vi "Launch Mask.vi"(4 "Pane Color":u32, 6 "Panel State":T1(ring)=enum."Standard", 8 "Error in":errorcluster caption="Error in (no error)", 9 "Bounds":T2, 10 "Panel Transparency":u8=60) -> (0 "Error out":errorcluster, 3 "reference out":refnum<vi>)   [LabVIEW 2016, in "Rectangle Mask.lvclass"]
uses:
  Classes/Rectangle Mask/Rectangle Mask.lvclass
  <vilib>/Utility/miscctls.llb/LVRectTypeDef.ctl
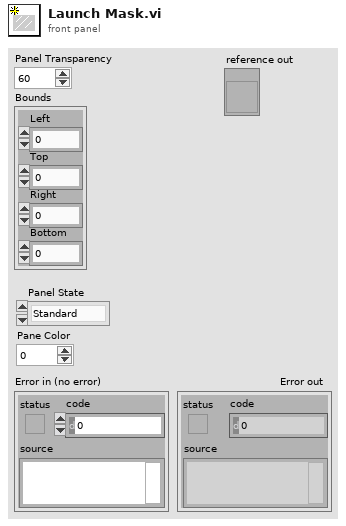
[diagram p1: front panel]
types:
  T1 = enum32{"Invalid", "Standard", "Closed", "Hidden", "Minimized", "Maximized"}
  T2 = typedef "LVRectTypeDef.ctl" = cluster{"Left":i16, "Top":i16, "Right":i16, "Bottom":i16}
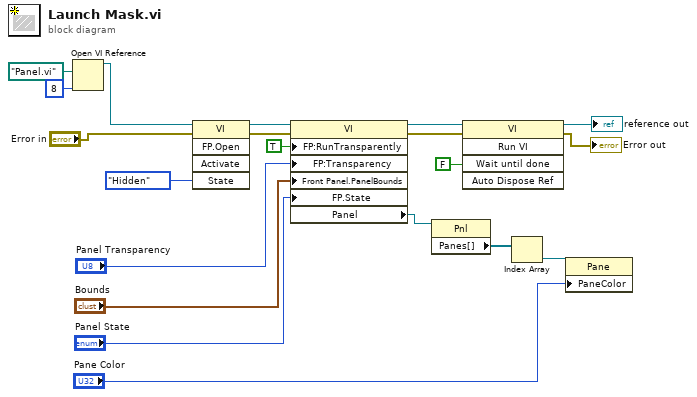
[diagram p0: block diagram]
diagram:
  n1 = Open VI Reference(vi path=path "Panel.vi", options=8) -> (vi reference=w9:refnum<vi>)  [unwired: 4 in, 1 out]
  n2 = invoke class="VI" method="FP.Open"(reference=w9, error in="Error in", "State"=T1."Hidden") -> (reference out=w16:refnum<vi>, error out=w15:errorcluster)  [unwired: 2 in, 3 out]
  n3 = property class="VI"(reference=w16, error in=w15, "FP:RunTransparently"=TRUE ("Front Panel Window:Run VI Transparently"), "FP:Transparency"="Panel Transparency", "Front Panel.PanelBounds"="Bounds", "FP.State"="Panel State") -> (reference out=w20:refnum<vi>, error out=w19:errorcluster, "Panel"=w4:refnum<vi>)
  n4 = property class="Pnl"(reference=w4) -> ("Panes[]"=w3:refnum<vi>[])  [unwired: 1 in, 2 out]
  n5 = invoke class="VI" method="Run VI"(reference=w20, error in=w19, "Wait until done"=FALSE ("Wait Until Done")) -> (reference out=→"reference out":refnum<vi>, error out=→"Error out":errorcluster)  [unwired: 2 in, 3 out]
  n6 = Index Array(array=w3) -> (element=w2:refnum<vi>)  [unwired: 1 in]
  n7 = property class="Pane"(reference=w2, "PaneColor"="Pane Color") -> ()  [unwired: 1 in, 2 out]
